vi "历史温度曲线.vi"() -> ()   [LabVIEW 2016, in "斯坦道通用流路CODmn.lvlib"]
uses:
  <vilib>/Utility/miscctls.llb/LVPointTypeDef.ctl
  <vilib>/Utility/miscctls.llb/LVRowAndColumnUnsignedTypeDef.ctl
  <vilib>/Utility/tdmsutil.llb/TDMSFileViewerLocalizedText.vi
panel:
  in  "参数下拉列表":u16(ring)
  in  "选项卡控件":enum32{"趋势图", "测试数据"}(tab)
  out "波形图":waveform(dbl)[](graph)
  out "显示值":string
  in  "多列列表框":i32(listbox)
  in  "列表框":i32(listbox)
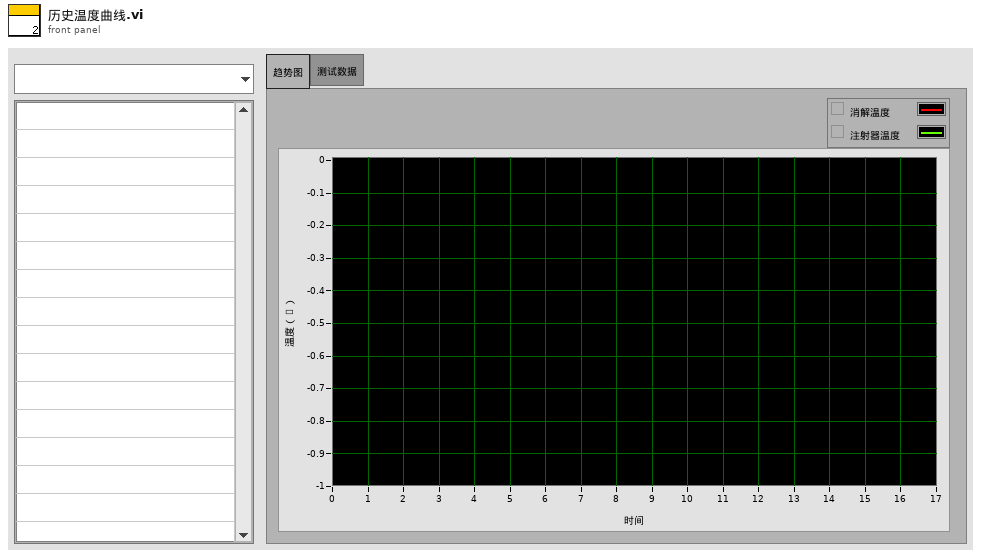
[diagram p1: front panel]
types:
  T1 = typedef "LVRowAndColumnUnsignedTypeDef.ctl" = cluster{"Row":u32, "Column":u32}
  T2 = typedef "LVPointTypeDef.ctl" = cluster{"Horizontal":i16, "Vertical":i16}
  T3 = typedef "SingleStepTestV3.lvlib/SingleStepTestV3.lvclass/仪器版本.ctl" = enum16{"A版", "B版", "A1版"}
  T4 = typedef "LVStringsAndValuesArrayTypeDef_U16.ctl" = cluster{"String":string, "Value":u16}[]
  T5 = typedef "LVPoint32TypeDef.ctl" = cluster{"Horizontal":i32, "Vertical":i32}
  T6 = typedef "Type Enum.ctl" = enum8{"Void", "I8", "I16", "I32", "I64", "U8", "U16", "U32", "U64", "Single Float", "Double Float", "Extended Float", "Single Complex", "Double Complex", "Extended Complex", "Enum I8 NEVER", "Enum I16 NEVER", "Enum I32 NEVER", "Enum I64 NEVER", "Enum U8", "Enum U16", "Enum U32", "Enum U64", "Single Float With Unit", "Double Float With Unit", "Extended Float With Unit", "Single Complex With Unit", "Double Complex With Unit", "Extended Complex With Unit", "boolU16", "Boolean", "String", "Handle", "Path", "Picture", "C String", "Pascal String", "Tag", "SubString", "Array", "SubArray", "Cluster", "Numeric Cluster", "Variant", "LV Variant", "Measure Data (waveform)", "Refnum", "ExtData", "function", "Typedef", "Poly VI", "bad wire", "LabVIEW Class Instance"}
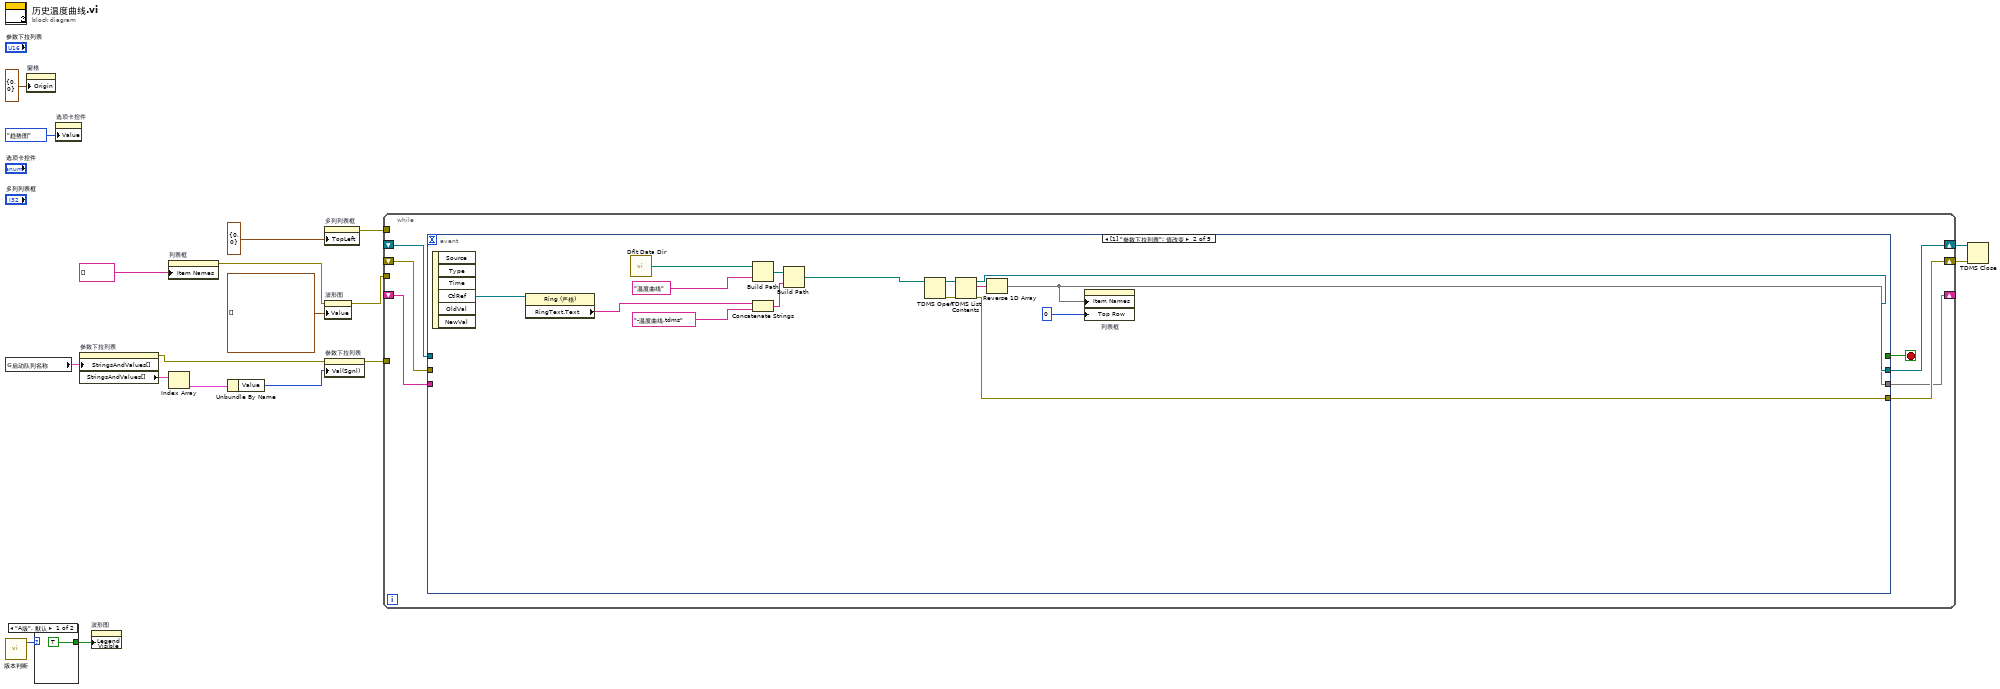
[diagram p0: block diagram]
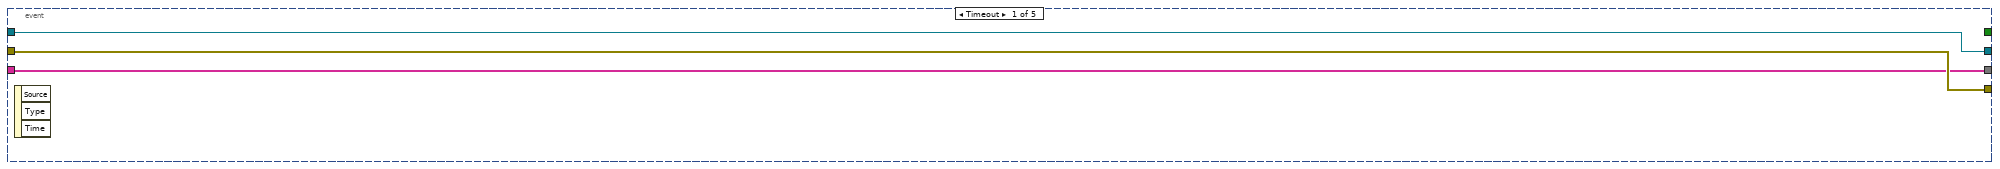
[diagram p3: hidden frame]
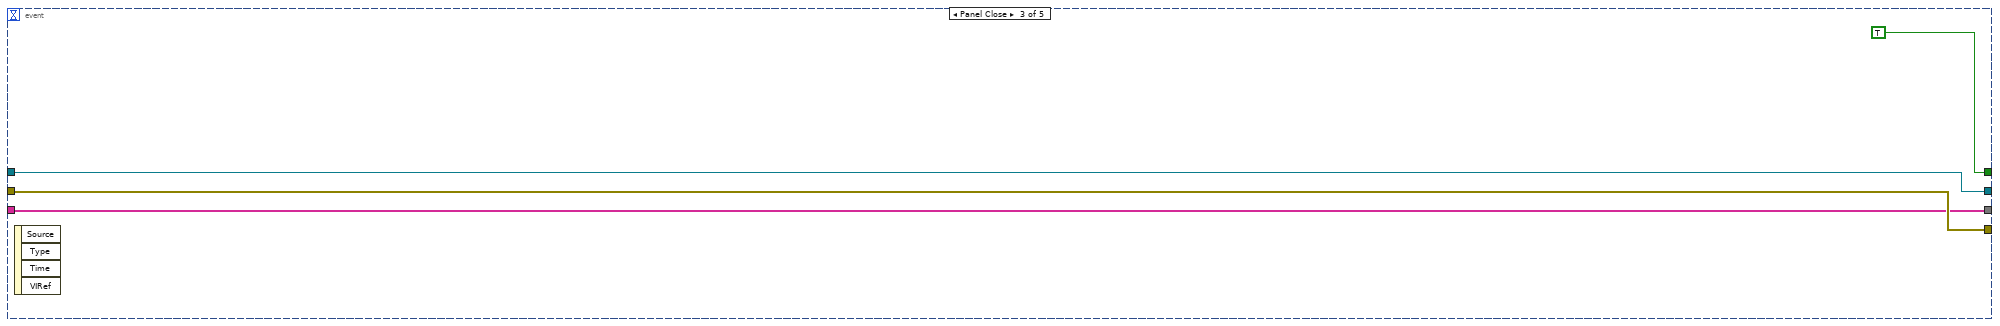
[diagram p4: hidden frame]
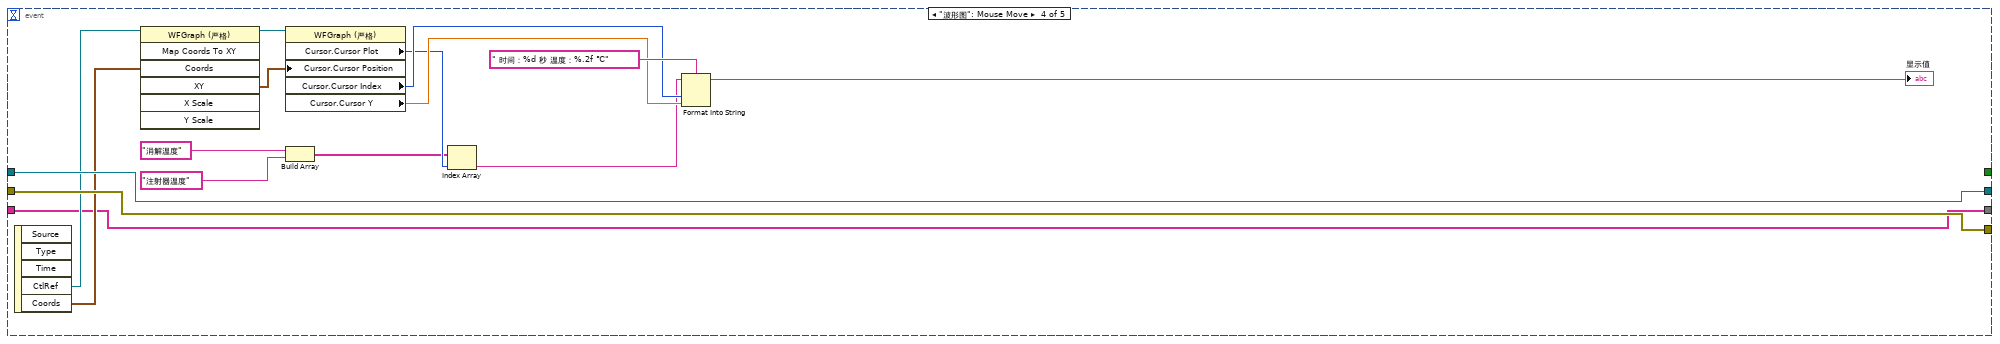
[diagram p5: hidden frame]
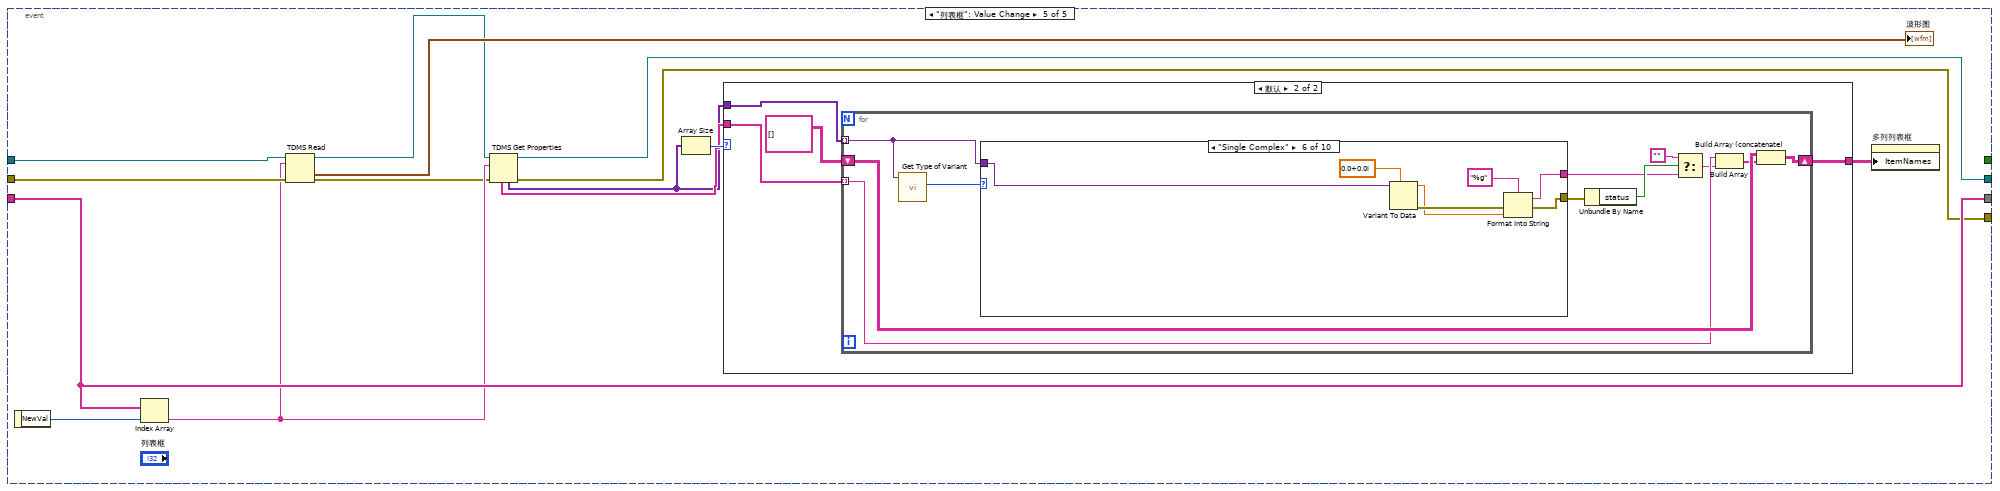
[diagram p6: hidden frame]
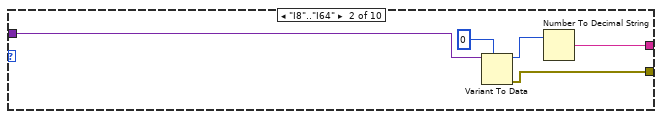
[diagram p9: hidden frame]
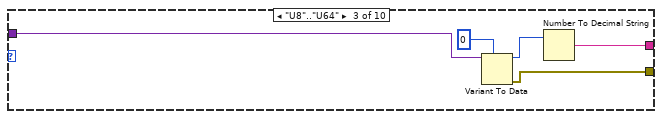
[diagram p10: hidden frame]
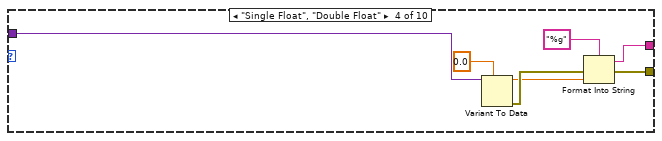
[diagram p11: hidden frame]
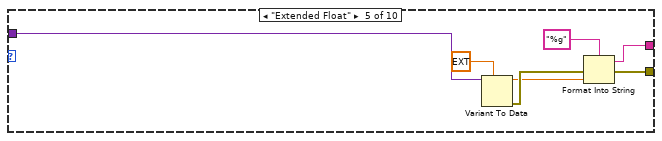
[diagram p12: hidden frame]
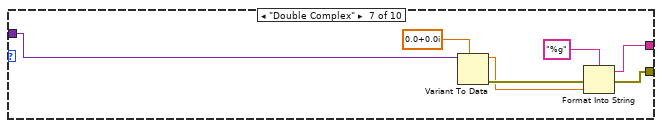
[diagram p13: hidden frame]
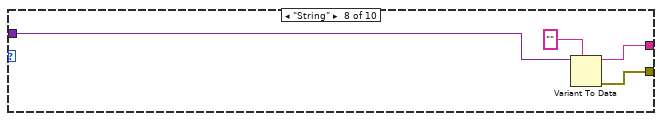
[diagram p14: hidden frame]
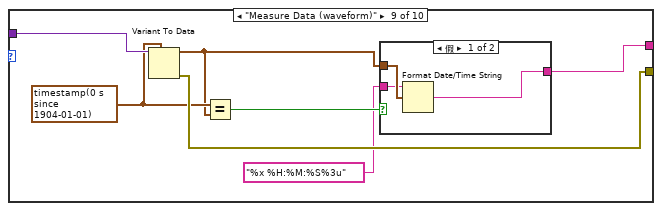
[diagram p15: hidden frame]
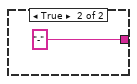
[diagram p16: hidden frame]
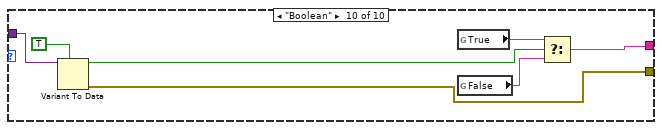
[diagram p17: hidden frame]
diagram:
  n1 = global read "model config var.vi" "启动队列名称"() -> (w6:cluster{"String":string, "Value":u16}[])
  n2 = call "版本判断.vi"() -> ("仪器版本"=w1:T3)  [unwired: 11 in]
  n3 = property on="窗格" class="Pane"("Origin"=T2 {"Horizontal"=0, "Vertical"=0} ("原点")) -> ()  [unwired: 2 in, 2 out]
  n4 = case shown="\"A版\", 默认" w1 {
    tunnel: [TRUE ("图例:曲线可见性复选框可见") _] -> w2
    frame "A版", Default {
    }
    frame "B版" {
    }
  }
  n5 = property on="选项卡控件" class="TabCtl (严格)"("Value"=enum32{"趋势图", "测试数据"}."趋势图" ("选项卡控件")) -> ()  [unwired: 2 in, 2 out]
  n6 = property on="参数下拉列表" class="Ring (严格)"("StringsAndValues[]"=w6) -> (error out=w9:errorcluster, "StringsAndValues[]"=w7:T4)  [unwired: 2 in, 1 out]
  n7 = property on="波形图" class="WFGraph (严格)"("Legend Visible"=w2) -> ()  [unwired: 2 in, 2 out]
  n8 = property on="列表框" class="LstBox (严格)"("Item Names"=string[] [] ("项名")) -> (error out=w15:errorcluster)  [unwired: 2 in, 1 out]
  n9 = Index Array(array=w7) -> (element=w8:cluster{"String":string, "Value":u16})  [unwired: 1 in]
  n10 = Unbundle By Name(w8) -> ("Value"=w10:u16)
  n11 = property on="多列列表框" class="MCListbox (严格)"("TopLeft"=T1 {"Row"=0, "Column"=0} ("左上可见单元格")) -> (error out=w4:errorcluster)  [unwired: 2 in, 1 out]
  n12 = property on="波形图" class="WFGraph (严格)"(error in=w15, "Value"=waveform(dbl)[] [] ("波形图")) -> (error out=w11:errorcluster)  [unwired: 1 in, 1 out]
  n13 = property on="参数下拉列表" class="Ring (严格)"(error in=w9, "Val(Sgnl)"=w10) -> (error out=w5:errorcluster)  [unwired: 1 in, 1 out]
  n14 = while {
    shift-right: [w24] -> w14
    shift-left: _ -> [w26]
    shift-right: [w23] -> w13
    shift-left: _ -> [w25]
    tunnel: w11 -> [_]
    shift-right: [w20] -> _
    shift-left: _ -> [w22]
    tunnel: w5 -> [_]
    tunnel: w4 -> [_]
    stop <- w21 stop-if-true
    n15 = event shown="[1] \"参数下拉列表\": 值改变" {
      selector: _ -> [_ _ _ _ _]
      dyn-events: _ -> [_ _ _ _ _]
      timeout: _ -> [_ _ _ _ _]
      tunnel: w26 -> [w29 _ w47 w61 w78]
      tunnel: w25 -> [w28 _ w46 w60 w77]
      tunnel: [w29 w37 w47 w61 w67] -> w24
      tunnel: [w28 w36 w46 w60 w66] -> w23
      tunnel: w22 -> [w27 _ w45 w49 w76]
      tunnel: [_ _ TRUE _ _] -> w21
      tunnel: [w27 w30 w45 w49 w76] -> w20
      event Timeout {
        n16 = event-data() -> ()  [unwired: 1 in, 3 out]
      }
      event "参数下拉列表": Value Change {
        n17 = event-data() -> ("CtlRef"=w35:refnum<vi>)  [unwired: 1 in, 5 out]
        n18 = property class="Ring (严格)"(reference=w35) -> ("RingText.Text"=w33:string)  [unwired: 1 in, 2 out]
        n19 = call <vilib>:"Dflt Data Dir.vi"() -> ("App:Default Data Directory"=w38:path)
        n20 = Build Path(base path=w38, name or relative path="温度曲线" ("名称或相对路径")) -> (appended path=w40:path)
        n21 = Concatenate Strings(w33, "-温度曲线.tdms" ("字符串")) -> (w32:string)
        n22 = Build Path(base path=w40, name or relative path=w32) -> (appended path=w41:path)
        n23 = TDMS Open(11:w41) -> (0:w43:errorcluster, 3:w42:refnum<k34>)  [unwired: 6 in]
        n24 = TDMS List Contents(4:w43, 7:w42) -> (0:w36:errorcluster, 2:w44:string[], 3:w37:refnum<k34>)  [unwired: 1 in, 1 out]
        n25 = Reverse 1D Array(array=w44) -> (reversed array=w30:string[])
        n26 = property on="列表框" class="LstBox (严格)"("Item Names"=w30, "Top Row"=0 ("顶行")) -> ()  [unwired: 2 in, 2 out]
      }
      event Panel Close {
        n27 = event-data() -> ()  [unwired: 1 in, 4 out]
      }
      event "波形图": Mouse Move {
        n28 = event-data() -> ("CtlRef"=w59:refnum<vi>, "Coords"=w58:T5)  [unwired: 1 in, 3 out]
        n29 = invoke on="调用节点" class="WFGraph (严格)" method="Map Coords To XY"(reference=w59, "Coords"=w58) -> (reference out=w56:refnum<vi>, "XY"=w64:cluster{"X":dbl, "Y":dbl})  [unwired: 5 in, 5 out]
        n30 = property on="属性节点" class="WFGraph (严格)"(reference=w56, "Cursor.Cursor Position"=w64) -> ("Cursor.Cursor Plot"=w54:i32, "Cursor.Cursor Index"=w62:i32, "Cursor.Cursor Y"=w55:dbl)  [unwired: 1 in, 2 out]
        n31 = Build Array("消解温度", "注射器温度") -> (w51:string[])
        n32 = Index Array(array=w51, index=w54) -> (element=w50:string)
        n33 = Format Into String(format string=" 时间：%d 秒 温度：%.2f ℃" ("格式字符串"), initial string=w50, w62, w55) -> (resulting string=→"显示值":string)  [unwired: 1 in, 1 out]
      }
      event "列表框": Value Change {
        n34 = event-data() -> ("NewVal"=w75:i32)  [unwired: 1 in]
        n35 = Index Array(array=w76, index=w75) -> (element=w69:string)
        n36 = TDMS Read(0:w78, 5:w69, 11:w77) -> (4:w70:refnum<k34>, 10:→"波形图":waveform(dbl)[], 15:w68:errorcluster)  [unwired: 5 in, 3 out]
        n37 = TDMS Get Properties(8:w68, 10:w69, 11:w70) -> (0:w66:errorcluster, 3:w67:refnum<k34>, 4:w71:variant[], 6:w72:string[])  [unwired: 3 in, 2 out]
        n38 = Array Size(array=w71) -> (size(s)=w73:i32)
        n39 = case shown="默认" w73 {
          tunnel: w72 -> [_ w82]
          tunnel: w71 -> [_ w81]
          tunnel: [_ w79] -> w65
          frame 0 {
          }
          frame Default {
            n40 = for {
              tunnel: w81 -> [w93] mode=indexing
              tunnel: w82 -> [w90] mode=indexing
              shift-right: [w91] -> w79
              shift-left: string[][] [] -> [w92]
              n41 = call <vilib>:"Get Type of Variant.vi"("Data In"=w93) -> ("Type Enum"=w89:T6)  [unwired: 9 in, 1 out]
              n42 = case shown="\"Single Complex\"" w89 {
                tunnel: w93 -> [_ w98 w103 w110 w117 w124 w131 w135 w142 w153]
                tunnel: [_ w95 w100 w107 w113 w120 w128 w133 w141 w152] -> w88
                tunnel: [_ w94 w99 w106 w112 w121 w127 w132 w140 w149] -> w86
                frame "Void", Default {
                }
                frame "I8".."I64" {
                  n43 = Variant To Data(type=i64 0 ("offset (0)"), Variant=w98) -> (data=w96:i64, error out=w95:errorcluster)  [unwired: 1 in]
                  n44 = Number To Decimal String(number=w96) -> (decimal integer string=w94:string)  [unwired: 1 in]
                }
                frame "U8".."U64" {
                  n45 = Variant To Data(type=u64 0 ("offset (0)"), Variant=w103) -> (data=w101:u64, error out=w100:errorcluster)  [unwired: 1 in]
                  n46 = Number To Decimal String(number=w101) -> (decimal integer string=w99:string)  [unwired: 1 in]
                }
                frame "Single Float", "Double Float" {
                  n47 = Variant To Data(type=0.0 ("offset (0)"), Variant=w110) -> (data=w104:dbl, error out=w108:errorcluster)  [unwired: 1 in]
                  n48 = Format Into String(format string="%g", error in=w108, w104) -> (resulting string=w106:string, error out=w107:errorcluster)  [unwired: 1 in]
                }
                frame "Extended Float" {
                  n49 = Variant To Data(type=ext 0.0 ("offset (0)"), Variant=w117) -> (data=w111:ext, error out=w114:errorcluster)  [unwired: 1 in]
                  n50 = Format Into String(format string="%g", error in=w114, w111) -> (resulting string=w112:string, error out=w113:errorcluster)  [unwired: 1 in]
                }
                frame "Single Complex" {
                  n51 = Variant To Data(type=csg 0.0+0.0i, Variant=w124) -> (data=w119:csg, error out=w122:errorcluster)  [unwired: 1 in]
                  n52 = Format Into String(format string="%g", error in=w122, w119) -> (resulting string=w121:string, error out=w120:errorcluster)  [unwired: 1 in]
                }
                frame "Double Complex" {
                  n53 = Variant To Data(type=cdb 0.0+0.0i, Variant=w131) -> (data=w126:cdb, error out=w129:errorcluster)  [unwired: 1 in]
                  n54 = Format Into String(format string="%g", error in=w129, w126) -> (resulting string=w127:string, error out=w128:errorcluster)  [unwired: 1 in]
                }
                frame "String" {
                  n55 = Variant To Data(type="" ("offset (0)"), Variant=w135) -> (data=w132:string, error out=w133:errorcluster)  [unwired: 1 in]
                }
                frame "Measure Data (waveform)" {
                  w139 = timestamp(0 s since 1904-01-01) ("offset (0)")
                  n56 = Variant To Data(type=w139, Variant=w142) -> (data=w138:timestamp, error out=w141:errorcluster)  [unwired: 1 in]
                  n57 = Equal?(x=w139, y=w138) -> (x = y?=w137:bool)
                  n58 = case shown="假" w137 {
                    tunnel: w138 -> [w145 _]
                    tunnel: [w144 "-" ("date/time string")] -> w140
                    tunnel: "%x %H:%M:%S%3u" ("time format string (%c)") -> [w143 _]
                    frame False {
                      n59 = Format Date/Time String(time format string (%c)=w143, seconds (now)=w145) -> (date/time string=w144:string)  [unwired: 1 in]
                    }
                    frame True {
                    }
                  }
                }
                frame "Boolean" {
                  n60 = Variant To Data(type=TRUE, Variant=w153) -> (data=w150:bool, error out=w152:errorcluster)  [unwired: 1 in]
                  n61 = global read "TDMSFileViewerLocalizedText.vi" "True"() -> (w147:string)
                  n62 = global read "TDMSFileViewerLocalizedText.vi" "False"() -> (w148:string)
                  n63 = Select(t=w147, s=w150, f=w148) -> (s? t:f=w149:string)
                }
              }
              n64 = Unbundle By Name(w88) -> ("status"=w87:bool)
              n65 = Select(t="", s=w87, f=w86) -> (s? t:f=w84:string)
              n66 = Build Array(w90, w84) -> (w83:string[])
              n67 = Build Array (concatenate)(w92, w83) -> (w91:string[][])
            }
          }
        }
        n68 = property on="多列列表框" class="MCListbox (严格)"("ItemNames"=w65) -> ()  [unwired: 2 in, 2 out]
      }
    }
  }
  n69 = TDMS Close(8:w13, 11:w14) -> ()  [unwired: 2 out]
